vi "WriteGlobal.vi"   [LabVIEW 2010]
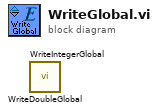
[diagram p0: block diagram]
diagram:
  n1 = call "WriteIntegerGlobal.vi"() -> ()  [unwired: 14 in, 2 out]
  n2 = call "WriteDoubleGlobal.vi"() -> ()  [unwired: 14 in, 2 out]
